vi "in out counter.vi"() -> ()   [LabVIEW 2022 SP3]
uses:
  <vilib>/DAQmx/create/channels.llb/DAQmx Create Channel (DI-Digital Input).vi
  <vilib>/DAQmx/miscellaneous.llb/DAQmx Fill In Error Info.vi
panel:
  out "IN ROOM":dbl
  out "OUT COUNT":dbl
  out "IN COUNT":dbl
  out "Boolean 2":bool
  in  "lines 2":tag
  in  "stop":bool
  out "Boolean":bool
  in  "lines":tag
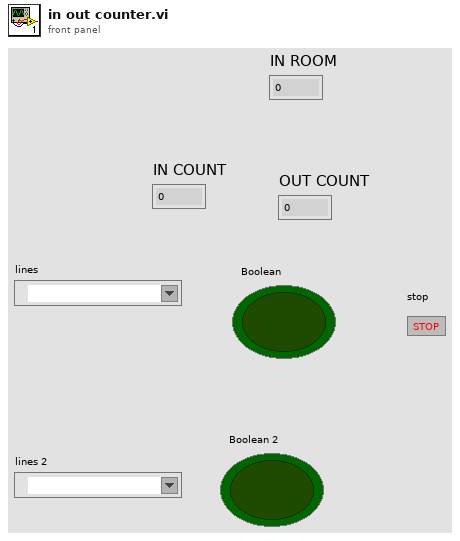
[diagram p1: front panel]
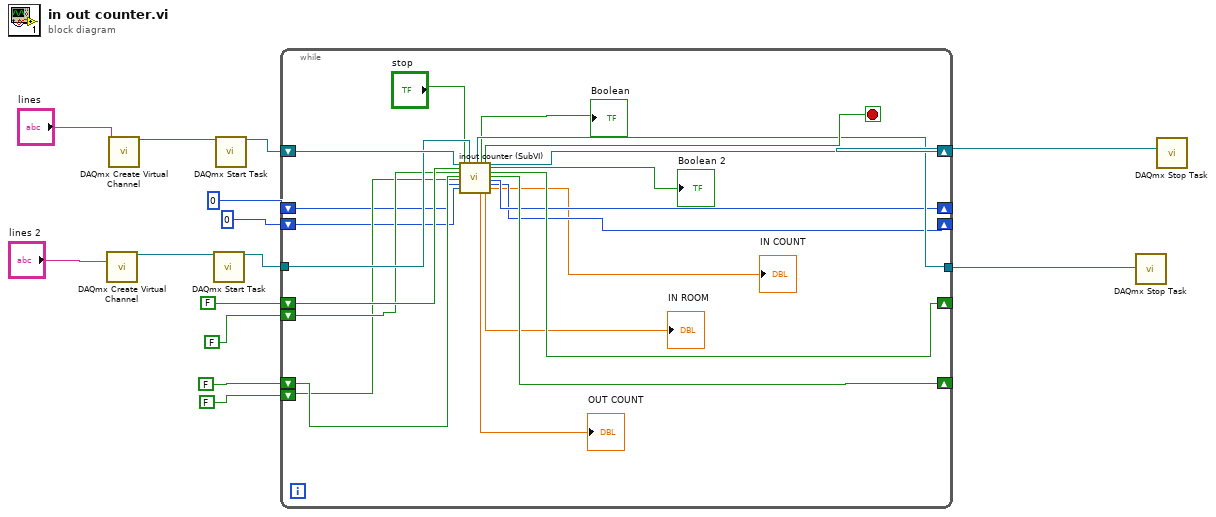
[diagram p0: block diagram]
diagram:
  n1 = call-poly <vilib>:"DAQmx Create Virtual Channel.vi"("lines"="lines 2") -> ("task out"=w10:refnum<k21>)  [unwired: 13 in, 1 out]
  n2 = call-poly <vilib>:"DAQmx Create Virtual Channel.vi"("lines"="lines") -> ("task out"=w14:refnum<k21>)  [unwired: 13 in, 1 out]
  n3 = call <vilib>:"DAQmx Start Task.vi"("task/channels in"=w10) -> ("task out"=w8:refnum<k21>)  [unwired: 13 in, 1 out]
  n4 = call <vilib>:"DAQmx Start Task.vi"("task/channels in"=w14) -> ("task out"=w13:refnum<k21>)  [unwired: 13 in, 1 out]
  n5 = while {
    shift-right: [w34] -> w12
    shift-left: w13 -> [w35]
    tunnel: w8 -> [w32]
    tunnel: [w31] -> w7
    shift-right: [w25] -> _
    shift-left: FALSE -> [w30]
    shift-right: [w24] -> _
    shift-left: FALSE -> [w28]
    shift-left: FALSE -> [w29]
    shift-left: FALSE -> [w27]
    shift-right: [w22] -> _
    shift-left: 0 -> [w26]
    shift-right: [w21] -> _
    shift-left: 0 -> [w23]
    stop <- w33 stop-if-true
    n6 = call "inout counter (SubVI).vi"("Refnum in"=w35, "Boolean 8"=w30, "Boolean 7"=w29, "Boolean 6"=w28, "Boolean 5"=w27, "Numeric 4"=w26, "Numeric 3"=w23, "stop in"="stop", "task in"=w32) -> ("task out"=w31:refnum<k21>, "Boolean"=→"Boolean":bool, "OUT COUNT"=→"OUT COUNT":dbl, "stop out"=w33:bool, "IN ROOM"=→"IN ROOM":dbl, "Refnum out"=w34:refnum<k21>, "Boolean 2"=→"Boolean 2":bool, "Boolean 4"=w25:bool, "Boolean 3"=w24:bool, "Numeric 2"=w22:i32, "Numeric"=w21:i32, "IN COUNT"=→"IN COUNT":dbl)  [unwired: 7 in]
  }
  n7 = call <vilib>:"DAQmx Stop Task.vi"("task/channels in"=w7) -> ()  [unwired: 13 in, 2 out]
  n8 = call <vilib>:"DAQmx Stop Task.vi"("task/channels in"=w12) -> ()  [unwired: 13 in, 2 out]
